vi "Platform System Time.vi"(8 "error in (no error)":errorcluster, 10 "System Time (12:59:42)":timestamp=timestamp(3346212582.1080246 s since 1904-01-01) format="%<%H:%M:%S>T", 11 "VISA resource name":refnum<visa-resource-name>) -> (0 "error out":errorcluster, 3 "VISA resource name out":refnum<visa-resource-name>)   [LabVIEW 2018, in "LTB-1.lvlib" / "3150.lvlib"]
doc: "The device has an internal clock and implements the SYSTem:TIME command to set the clock time over the interface."
uses:
  3150.lvlib
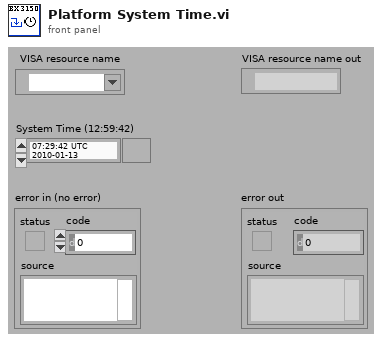
[diagram p1: front panel]
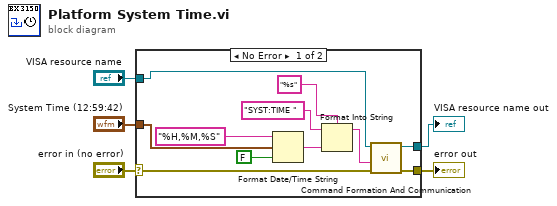
[diagram p0: block diagram]
diagram:
  n1 = case shown="No Error" "error in (no error)" {
    selector: "error in (no error)" -> [w15 w17]
    tunnel: "VISA resource name" -> [w16 w18]
    tunnel: [w13 w18] -> w4
    tunnel: [w14 w17] -> w3
    tunnel: "System Time (12:59:42)" -> [w7 _]
    frame No Error {
      n2 = Format Date/Time String(time format string (%c)="%H,%M,%S", seconds (now)=w7, UTC format=FALSE) -> (date/time string=w6:string)
      n3 = Format Into String(format string="%s", initial string="SYST:TIME " ("Command"), w6) -> (resulting string=w10:string)  [unwired: 1 in, 1 out]
      n4 = call "Command Formation And Communication.vi"("error in (no error)"=w15, "Command"=w10, "VISA resource name"=w16) -> ("error out"=w14:errorcluster, "VISA resource name out"=w13:refnum<visa-resource-name>)  [unwired: 1 in, 6 out]
    }
    frame Error {
    }
  }
  "VISA resource name out" <- w4
  "error out" <- w3
